vi "Replace NaN with 0 in temp.vi"(7 "Temperature in":dbl) -> (8 "Temperature out":dbl)   [LabVIEW 2011]
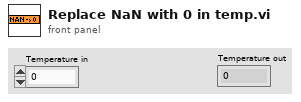
[diagram p1: front panel]
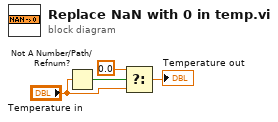
[diagram p0: block diagram]
diagram:
  n1 = Not A Number/Path/Refnum?(number/path/refnum="Temperature in") -> (NaN/Path/Refnum?=w1:bool)
  n2 = Select(t=0.0, s=w1, f="Temperature in") -> (s? t:f=→"Temperature out":dbl)
